vi "DAQ 1SDI v01.vi"() -> ()   [LabVIEW 2013]
uses:
  <instrlib>/niScope/Controls/niScope vertical coupling.ctl
  Global VIs/shotnoise.vi
panel:
  out "Signal 2":dbl[](graph)
  out "Signal 1":dbl[](graph)
  out "error out":errorcluster caption="error out final"
  out "error out TDMS":errorcluster caption="error out"
  in  "stop":bool
  in  "?":T1(tab)
  out "Video bandwidth (Hz)":dbl=3333.3333333333335
  in  "DAQ Card":refnum<k15>="PXI2Slot2"
  in  "Minimum sample rate (S/s)":dbl=100000000.0 format="%#_6p"
  in  "Reference position":dbl(slide)=50.0 scale=0.0..100.0
  in  "max time (s)":dbl=10.0 caption="Time to run (s)"
  in  "Channel parameters":T3(array[cluster])=[{"Channel name"="0", "Input impedance (Ohms)"=2, "Maximum input frequency (Hz)"=30000000.0, "vertical coupling"=1, "Probe attenuation"=1.0, "Vertical range (V)"=0.2, "Vertical offset"=0.0, "channel enabled"=TRUE}, {"Channel name"="1", "Input impedance (Ohms)"=2, "Maximum input frequency (Hz)"=30000000.0, "vertical coupling"=1, "Probe attenuation"=1.0, "Vertical range (V)"=0.2, "Vertical offset"=0.0, "channel enabled"=TRUE}] {"Input impedance (Ohms)" items=["1 mega ohm"=0, "50 ohms"=2]; "Maximum input frequency (Hz)" format="%#_6p"; "vertical coupling" items=["AC", "DC", "Ground"]}
  in  "IIR filter specifications":T4={"Topology"=enum."Butterworth", "Type"=enum."Bandpass", "Order"=6, "Lower Fc"=2700000.0, "Upper Fc"=3100000.0, "PB Ripple"=1.0, "SB Attenuation"=60.0} {"PB Ripple" format="%0.2f"; "SB Attenuation" format="%0.2f"; "Lower Fc" format="%0.2p"; "Upper Fc" format="%0.2p"}
  out "Number of samples":i32=30000 format="%.0p"
  out "Variance 1 normalised to SNL":dbl(graph)=-16.0816956179939
  out "Conditional variance":dbl(graph)=0.024487105953063568
  in  "Shot noise start":bool
  out "Variance 2 normalised to SNL":dbl(graph)=-15.053649945243023
  in  "reset sn":bool
  out "SN":dbl[](array[numeric])=[0.0004701240049675991, 0.00028595268124144543]
  out "SN loop count":i64=74
  out "covariance":dbl(graph)=-0.002260946442750242
  out "Conditional variance 2":dbl(graph)=0.024487105953063568
  in  "Record Data":bool
  in  "File location":path=path "C:/Documents and Settings/QIM/My Documents/July 2010 data"
  in  "Type of measurement":u16
  out "Parameters values file":string="PARAMETERS VALUES\r\rFriday, 6 August 2010\r4:33 PM\r\rMaster ch 0 <-> HD1 AC a-b\nMaster ch 1 <-> HD2 AC a-b\n\r\r\r\rSample rate : \rMaster : 100.000000E+6 Samples per second\rNumber of samples :\rMaster ch 0 : 30.000000E+3\rMaster ch 1 : 30.000000E+3\rFiles names : \r9th_july_what_sqz_ParametersValues_30000.txt\r9th_july_what_sqz_mch0_30000.txt\r9th_july_what_sqz_mch1_30000.txt\r9th_july_what_sqz_mch01_60000.txt\r"
  in  "File root name":string="9th_july_what"
  in  "Number of samples":i32=30000 format="%.0p"
  out "Loop count":i32
  out "Actual samples acquired in waveform, ch 0":i32=30000
  out "Actual samples acquired in waveform, ch 1":i32=30000
  in  "File Name":path=path "C:/Documents and Settings/QIM/My Documents/LabVIEW Data/111016-discord-gain9-seed40-3/ele-0000mV-d0150mV-g9-s40.lvm"
  # "set to -1 to fetch all available samples"
  # "Variance won't be displayed until shot noise is taken"
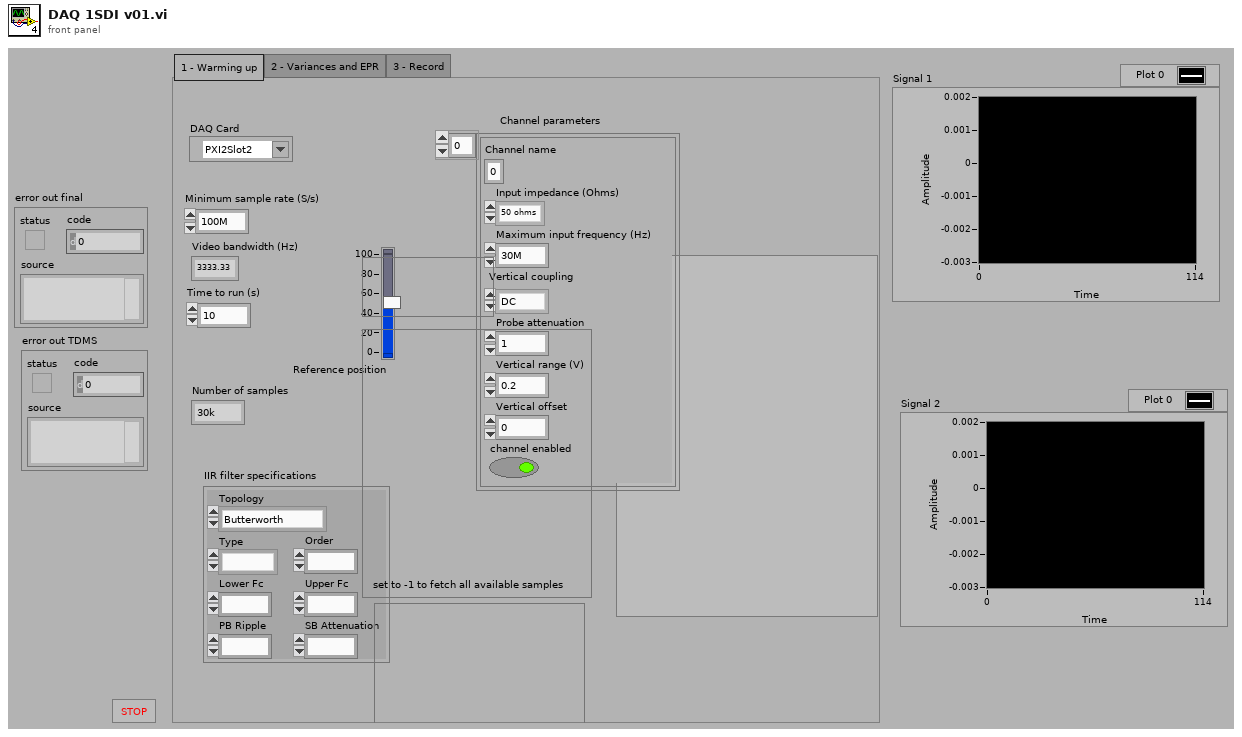
[diagram p1: front panel]
types:
  T1 = enum32{"1 - Warming up", "2 - Variances and EPR", "3 - Record"}
  T2 = typedef "niScope vertical coupling.ctl" = i32
  T3 = cluster{"Channel name":string, "Input impedance (Ohms)":u32, "Maximum input frequency (Hz)":dbl, "vertical coupling":T2, "Probe attenuation":dbl, "Vertical range (V)":dbl, "Vertical offset":dbl, "channel enabled":bool}[]
  T4 = cluster{"Topology":enum16{"Off", "Butterworth", "Chebyshev", "Inverse Chebyshev", "Elliptic", "Bessel"}, "Type":enum16{"Lowpass", "Highpass", "Bandpass", "Bandstop"}, "Order":i32, "Lower Fc":dbl, "Upper Fc":dbl, "PB Ripple":dbl, "SB Attenuation":dbl}
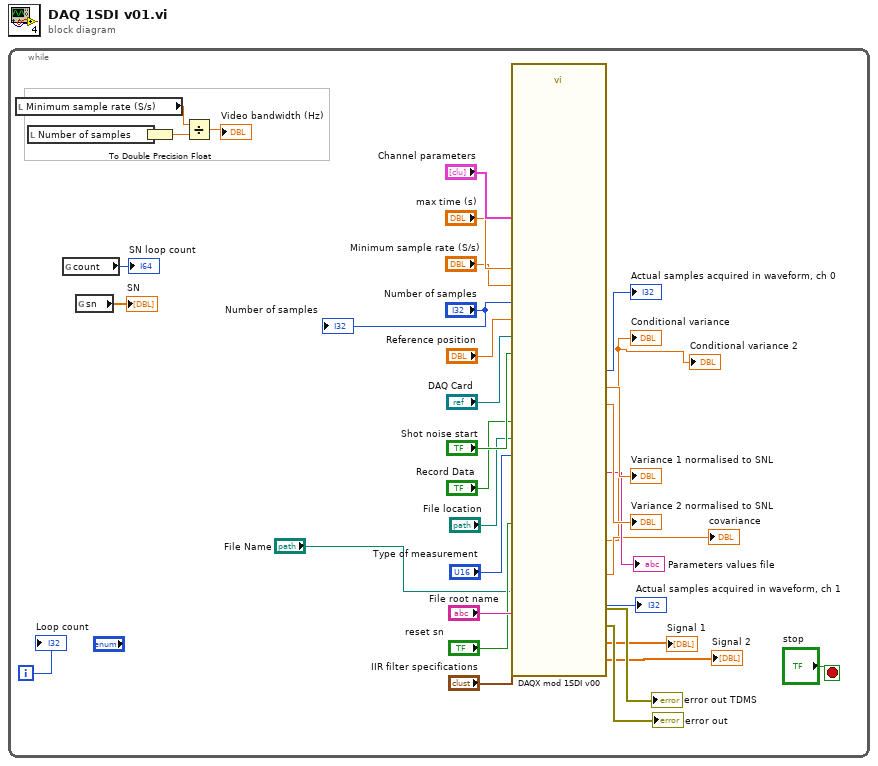
[diagram p0: block diagram]
diagram:
  n1 = while {
    i -> [w12]
    stop <- "stop" stop-if-true
    n2 = local read "Minimum sample rate (S/s)"() -> (w31:dbl)
    n3 = local read "Number of samples"() -> (w33:i32)
    n4 = global read "shotnoise.vi" "count"() -> (→"SN loop count":i64)
    n5 = global read "shotnoise.vi" "sn"() -> (→"SN":dbl[])
    n6 = To Double Precision Float(number=w33) -> (double precision float=w30:dbl)
    n7 = Divide(x=w31, y=w30) -> (x/y=→"Video bandwidth (Hz)":dbl)
    n8 = call "DAQX mod 1SDI v00.vi"("resource name"="DAQ Card", "Record Data"="Record Data", "numSamples"="Number of samples", "max time (s)"="max time (s)", "min sample rate"="Minimum sample rate (S/s)", "File location"="File location", "reference position"="Reference position", "IIR filter specifications"="IIR filter specifications", "Type of\nmeasurement"="Type of measurement", "Name root"="File root name", "File Name"="File Name", "channel parameters"="Channel parameters", "Shot noise start"="Shot noise start", "reset sn"="reset sn") -> ("Signal 1"=→"Signal 1":dbl[], "conditional variance"=→"Conditional variance" →"Conditional variance 2":dbl, "error out TDMS"=→"error out TDMS":errorcluster, "covariance"=→"covariance":dbl, "Variance 2 normalised to SNL"=→"Variance 2 normalised to SNL":dbl, "Signal 2"=→"Signal 2":dbl[], "Parameters values file"=→"Parameters values file":string, "Variance 1 normalised to SNL"=→"Variance 1 normalised to SNL":dbl, "actualSamples 0"=→"Actual samples acquired in waveform, ch 0":i32, "actualSamples 1"=→"Actual samples acquired in waveform, ch 1":i32, "error out"=→"error out":errorcluster)  [unwired: 2 in, 1 out]
    "Loop count" <- w12
    "Number of samples" <- "Number of samples"
  }
